vi "Generate Configuration.vi"(6 "Starting Address Offset":u16 format="%04x", 7 "Virtual Memory Unit in":refnum<class "Virtual Memory Unit.lvclass">, 8 "error in (no error)":errorcluster, 11 "Bus Monitor in":refnum<class "Bus Monitor.lvclass">) -> (0 "error out":errorcluster, 2 "Parameter List":string[](array[string]), 3 "Bus Monitor out":refnum<class "Bus Monitor.lvclass">, 4 "Next Address Offset":u16 format="%04x", 5 "Virtual Memory Unit out":refnum<class "Virtual Memory Unit.lvclass">)   [LabVIEW 2020, in "BCI-1553 API.lvlib" / "Bus Monitor.lvclass"]
uses:
  Bus Monitor.lvclass
  Dependencies/Virtual Memory Unit/Virtual Memory Unit.lvclass
  Bus Monitor.lvclass/Bus Monitor.ctl
  Dependencies/Registry/Registry.lvclass/Registry.ctl
  Dependencies/Registry/Registry.lvclass
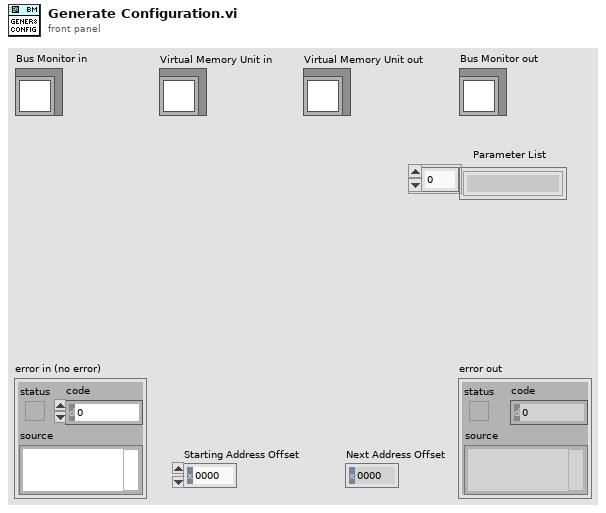
[diagram p1: front panel]
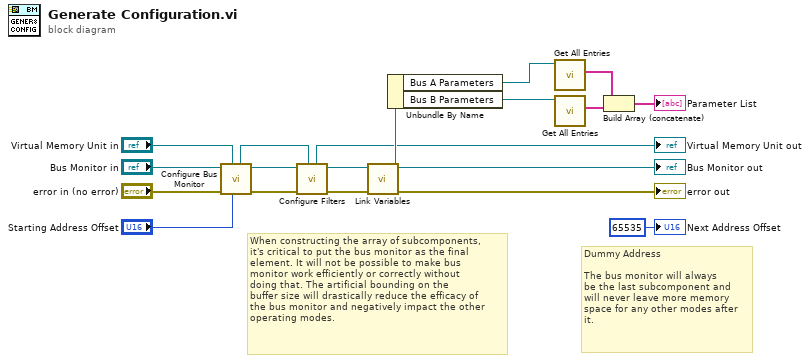
[diagram p0: block diagram]
diagram:
  # "Dummy Address\n\nThe bus monitor will always\nbe the last subcomponent and\nwill never leave more memory\nspace for any other modes after\nit."
  # "When constructing the array of subcomponents,\nit's critical to put the bus monitor as the final \nelement. It will not be possible to make bus \nmonitor work efficiently or correctly without\ndoing that. The artificial bounding on the \nbuffer size will drastically reduce the efficacy of\nthe bus monitor and negatively impact the other\noperating modes."
  n1 = call "Configure Bus Monitor.vi"("Starting Address Offset"="Starting Address Offset", "Virtual Memory Unit in"="Virtual Memory Unit in", "error in (no error)"="error in (no error)", "Bus Monitor in"="Bus Monitor in") -> ("error out"=w11:errorcluster, "Bus Monitor out"=w13:refnum<class "Bus Monitor.lvclass">, "Virtual Memory Unit out"=w4:refnum<class "Virtual Memory Unit.lvclass">)  [unwired: 5 in]
  n2 = call "Configure Filters.vi"("Virtual Memory Unit in"=w4, "error in (no error)"=w11, "Bus Monitor in"=w13) -> ("error out"=w10:errorcluster, "Bus Monitor out"=w14:refnum<class "Bus Monitor.lvclass">, "Virtual Memory Unit out"=→"Virtual Memory Unit out":refnum<class "Virtual Memory Unit.lvclass">)  [unwired: 6 in]
  n3 = call "Link Variables.vi"("error in (no error)"=w10, "Bus Monitor in"=w14) -> ("error out"=→"error out":errorcluster, "Bus Monitor out"=w5:refnum<class "Bus Monitor.lvclass">)  [unwired: 8 in]
  "Bus Monitor out" <- w5
  n4 = Unbundle By Name(w5) -> ("Bus A Parameters"=w8:refnum<class "Registry.lvclass">, "Bus B Parameters"=w7:refnum<class "Registry.lvclass">)
  n5 = call "Get All Entries.vi"("Registry in"=w8) -> ("Keys"=w17:string[])  [unwired: 8 in, 2 out]
  n6 = call "Get All Entries.vi"("Registry in"=w7) -> ("Keys"=w18:string[])  [unwired: 8 in, 2 out]
  n7 = Build Array (concatenate)(w17, w18) -> (→"Parameter List":string[])
  "Next Address Offset" <- u16 65535 ("Next Address Offset")
